vi "SwissSPAD Live_Image Histogram.vi"() -> ()   [LabVIEW 2021]
uses:
  Histograms/Histogram Bin Position.ctl
  SwissSPAD Live_Internal Data List.ctl
  SwissSPAD Live_Settings List.ctl
  SwissSPAD Live_Image Display Options.ctl
  Calc/Conditional Add 1.llb/Conditional Add 1 [I32].vi
  3eb8dcdc-dfa2-4210-84d8-37bed86b0045.vi/929807a6-00f9-4258-af09-20dfd637e3ca.vi
  3eb8dcdc-dfa2-4210-84d8-37bed86b0045.vi/52c6b4fa-501b-4af0-803b-8bab516ca5d3.vi
  3eb8dcdc-dfa2-4210-84d8-37bed86b0045.vi/d7237e10-35ab-4bcb-a0c6-4883c3f4c990.vi
  3eb8dcdc-dfa2-4210-84d8-37bed86b0045.vi/5fb5dd96-3b97-4592-ba56-58181c8e7105.vi
  3eb8dcdc-dfa2-4210-84d8-37bed86b0045.vi/8e13a849-a393-4484-9968-4af7b25c38d7.vi
  GUI/Dialog Window with Option.vi
  <vilib>/Analysis/baseanly.llb/Std Deviation and Variance.vi
  <vilib>/Utility/error.llb/Error Cluster From Error Code.vi
  Variant/Variant to Data/Variant to Data.lvlib
panel:
  in  "Cursor Update (Hidden)":bool
  in  "Stop (Hidden)":bool
  out "Image Histogram":cluster{"Axis":dbl[], "Histogram":dbl[]}(graph)
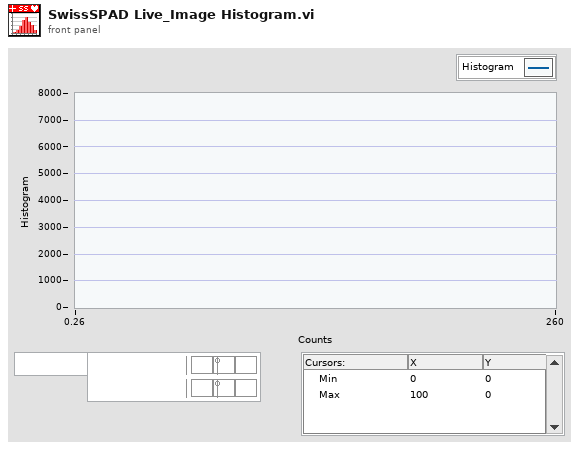
[diagram p1: front panel]
types:
  T1 = typedef "Histogram Bin Position.ctl" = enum16{"Left", "Center", "Right"}
  T2 = cluster{"Bin Size":dbl, "Min Value":dbl, "Max Value":dbl, "Filter NaN & Infinite Values":bool, "Frequency Plot":bool, "Align Bins":bool, "Bin Location":T1, "Project Outside Values":bool, "Max Histogram Size":i32}
  T3 = typedef "SwissSPAD Live_Internal Data List.ctl" = enum16{"Number of pending file saving tasks", "File Saving Tasks Information", "Current Image ROI Information", "# FPGA Reset Attempts", "Histogram Cursor Locations", "Histogram Window is Open"}
  T4 = typedef "SwissSPAD Live_Settings List.ctl" = enum16{"FPGA:Bottom Half", "FPGA:Top Half", "FPGA:Bottom Bitfile Path", "FPGA:Top Bitfile Path", "FPGA:Bottom Bitstream Version", "FPGA:Top Bitstream Version", "FPGA:Auto Reset FPGA", "FPGA:Bottom FPGA Serial Number", "FPGA:Top FPGA Serial Number", "FPGA:Detector PCB Version", "Acquisition Parameters:Microlens", "Acquisition Parameters:SS2 DAQ Parameters", "Acquisition Parameters:Gate Configuration Array", "Acquisition Parameters:SS3 DAQ Parameters", "Acquisition Parameters:Buffer Size (# 8-bit Gates)", "File Information:File Information", "File Information:# Datasets in Series", "File Information:Scrambled File Flag", "File Information:SS3 Gate Slip Correction", "File Information:SS3 Hot Pixel Mismatch Detection", "File Information:Delay between Datasets", "File Information:Save Sum of All Gates Preview", "Image Parameters:Image ROI Information", "Image Parameters:Image Binning Options", "Image Parameters:SS3 Displayed Image", "Image Parameters:Image Display Options", "Image Parameters:Use Histogram Cursors", "Image Parameter:FPGA Data to Display", "UI Settings:Histogram Bins Number", "UI Settings:Histogram Bin Size", "UI Settings:Use Image Display Options", "UI Settings:Verbose Settings", "UI Settings:Verbose Saving"}
  T5 = typedef "SwissSPAD Live_Image Display Options.ctl" = cluster{"Remove Screamers":bool, "Delta":sgl, "Equalize Histogram":bool, "Percentile":sgl, "Hot Pixel Mask Image":path, "Use Hot Pixel Mask":bool}
  T6 = typedef "Array Statistics.ctl" = cluster{"Mean":dbl, "Standard Deviation":dbl, "Max":dbl, "Min":dbl}
  T7 = typedef "LVCursorListTypeDef.ctl" = cluster{"Name":string, "Color":u32, "Style":u8, "Point Style":u8, "Name Visible":bool, "Allow Drag":bool, "Cursor Mode":u32, "Plot":i32, "Index":i32, "Position":cluster{"X":dbl, "Y":dbl}, "X Scale":u32, "Y Scale":u32, "Watch Plots":i32[], "Watch All Plots":bool, "Plot Area":i32, "Label Offset":cluster{"X":dbl, "Y":dbl}}[]
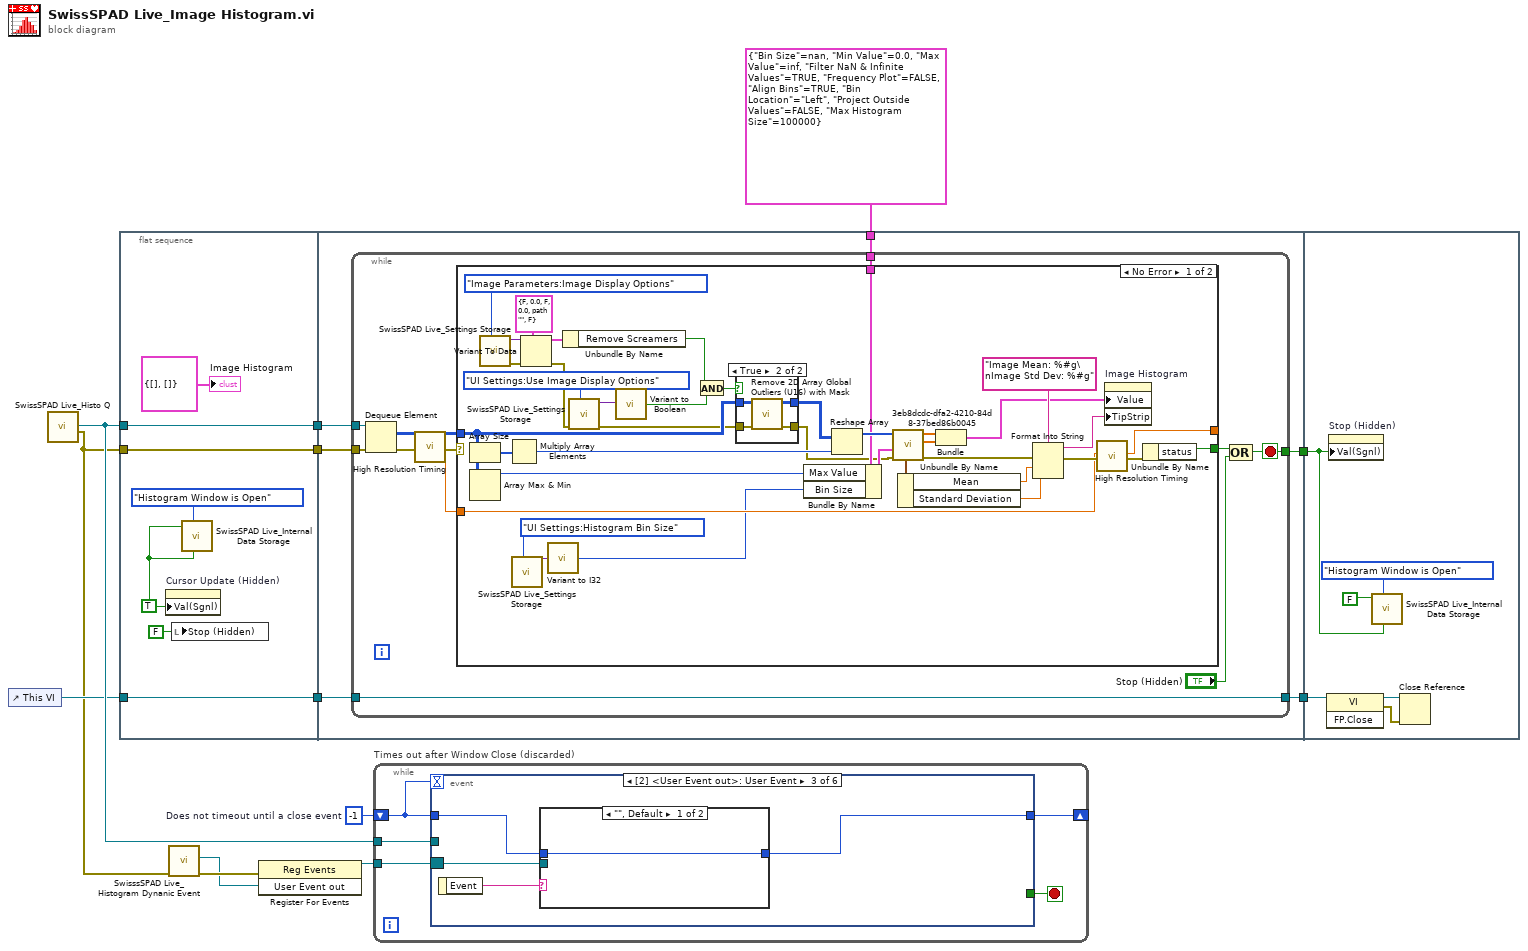
[diagram p0: block diagram]
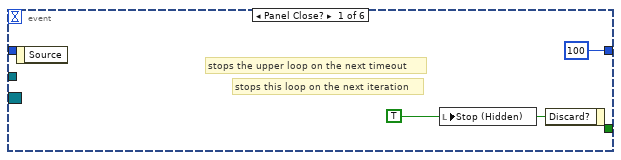
[diagram p2: hidden frame]
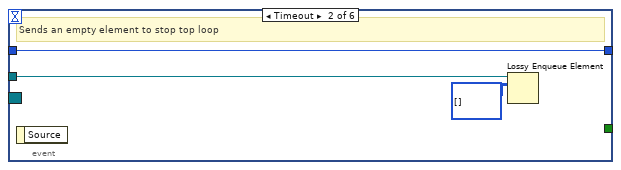
[diagram p3: hidden frame]
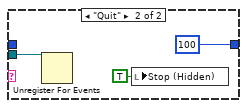
[diagram p4: hidden frame]
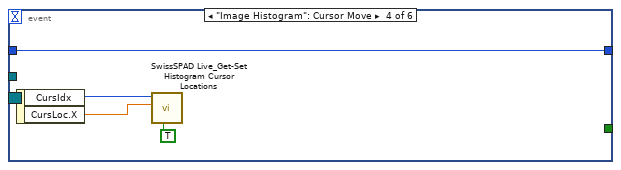
[diagram p5: hidden frame]
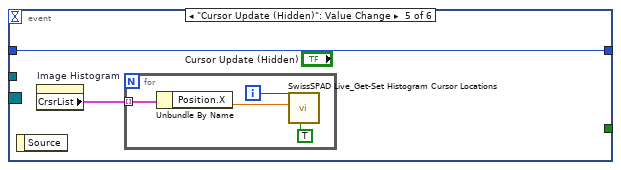
[diagram p6: hidden frame]
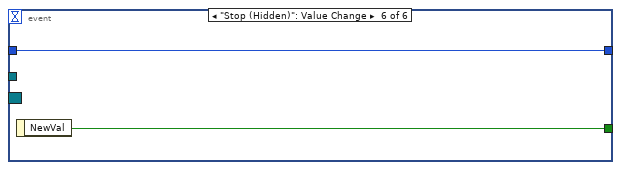
[diagram p7: hidden frame]
diagram:
  w11 = -1  # Does not timeout until a close event
  n1 = control-ref of="This VI"() -> (w6:refnum<vi>)
  n2 = call "SwissSPAD Live_Histo Q.vi"() -> ("error out"=w1:errorcluster, "SS2 Live Histo Q"=w8:refnum<queue>)  [unwired: 6 in]
  n3 = flat-sequence {
    tunnel: [w19] -> w10
    tunnel: w8 -> [w19]
    tunnel: [w18] -> w9
    tunnel: w1 -> [w18]
    tunnel: [w17] -> w7
    tunnel: w6 -> [w17]
    tunnel: [w26] -> w13
    tunnel: [w22] -> w12
    tunnel: w10 -> [w25]
    tunnel: w9 -> [w24]
    tunnel: w7 -> [w23]
    tunnel: T2 {"Bin Size"=nan, "Min Value"=0.0, "Max Value"=inf, "Filter NaN & Infinite Values"=TRUE, "Frequency Plot"=FALSE, "Align Bins"=TRUE, "Bin Location"=enum."Left", "Project Outside Values"=FALSE, "Max Histogram Size"=100000} ("Histogram Options") -> [w21]
    tunnel: w13 -> [w83]
    tunnel: w12 -> [w87]
    frame #0 {
      w16 = TRUE ("Value (Signaling)")
      n4 = property on="Cursor Update (Hidden)" class="Bool (strict)"("Val(Sgnl)"=w16) -> ()  [unwired: 2 in, 2 out]
      n5 = local write "Stop (Hidden)"(FALSE ("Stop")) -> ()
      n6 = call "SwissSPAD Live_Internal Data Storage.vi"("Get(F)/Set"=w16, "SS2 Live Data"=SwissSPAD_Live_Internal_Data_List."Histogram Window is Open", "Variant"=w16) -> ()  [unwired: 6 in, 3 out]
      "Image Histogram" <- cluster{"Axis":dbl[], "Histogram":dbl[]} {"Axis"=[], "Histogram"=[]} ("Image Histogram")
    }
    frame #1 {
      n7 = while {
        tunnel: [w33] -> w26
        tunnel: w25 -> [w32]
        tunnel: w24 -> [w31]
        tunnel: w23 -> [w30]
        tunnel: [w30] -> w22
        tunnel: w21 -> [w27]
        stop <- w33 stop-if-true
        n8 = Dequeue Element(queue=w32, error in (no error)=w31) -> (element=w36:u16[][], error out=w37:errorcluster)  [unwired: 1 in, 2 out]
        n9 = call "High Resolution Timing.vi"("Error In"=w37) -> ("elapsed (relative) seconds"=w28:dbl, "Error Out"=w29:errorcluster)  [unwired: 16 in, 1 out]
        n10 = case shown="No Error" w29 {
          tunnel: w36 -> [w45 _]
          tunnel: [w74 _] -> w35
          tunnel: w28 -> [w58 _]
          tunnel: [w57 _] -> _
          tunnel: w27 -> [w56 _]
          frame No Error {
            n11 = Array Size(array=w45) -> (size(s)=w73:i32[])
            n12 = Array Max & Min(array=w45) -> (max value=w61:u16)  [unwired: 3 out]
            n13 = call "SwissSPAD Live_Settings Storage.vi"("Settings List"=SwissSPAD_Live_Settings_List."Image Parameters:Image Display Options") -> ("Error Out"=w50:errorcluster, "Variant Data out"=w51:variant)  [unwired: 9 in]
            n14 = Multiply Array Elements(1:w73) -> (0:w72:i32)
            n15 = call "SwissSPAD Live_Settings Storage.vi"("Settings List"=SwissSPAD_Live_Settings_List."UI Settings:Histogram Bin Size") -> ("Variant Data out"=w54:variant)  [unwired: 9 in, 1 out]
            n16 = Variant To Data(error in=w50, type=T5 {"Remove Screamers"=FALSE, "Delta"=0.0, "Equalize Histogram"=FALSE, "Percentile"=0.0, "Hot Pixel Mask Image"=path "", "Use Hot Pixel Mask"=FALSE} ("Image Display Options"), Variant=w51) -> (data=w48:T5, error out=w43:errorcluster)
            n17 = call "Variant to I32.vi"("Variant"=w54) -> ("Value"=w38:i32)  [unwired: 8 in]
            n18 = Unbundle By Name(w48) -> ("Remove Screamers"=w47:bool)
            n19 = call "SwissSPAD Live_Settings Storage.vi"("Settings List"=SwissSPAD_Live_Settings_List."UI Settings:Use Image Display Options", "Error In"=w43) -> ("Error Out"=w40:errorcluster, "Variant Data out"=w42:variant)  [unwired: 8 in]
            n20 = call "Variant to Boolean.vi"("Variant"=w42) -> ("Value"=w41:bool)  [unwired: 8 in]
            n21 = And(x=w47, y=w41) -> (x .and. y?=w46:bool)
            n22 = case shown="True" w46 {
              tunnel: [w77 w81] -> w53
              tunnel: w40 -> [w76 w80]
              tunnel: w45 -> [w77 w79]
              tunnel: [w76 w78] -> w39
              frame False {
              }
              frame True {
                n23 = call "Remove 2D Array Global Outliers (U16) with Mask.vi"("Error In"=w80, "2D Array in"=w79) -> ("Error Out"=w78:errorcluster, "2D Array out"=w81:u16[][])  [unwired: 6 in, 2 out]
              }
            }
            n24 = Bundle By Name(cluster=w56, "Max Value"=w61, "Bin Size"=w38) -> (w60:T2)
            n25 = Reshape Array(w53, w72) -> (w71:u16[])
            n26 = call "3eb8dcdc-dfa2-4210-84d8-37bed86b0045.vi"("Error In"=w39, "Histogram Options"=w60, "Array"=w71) -> ("Error Out"=w70:errorcluster, "Array Statistics"=w69:T6, "Histogram"=w65:dbl[], "Axis"=w66:dbl[])  [unwired: 4 in, 1 out]
            n27 = Unbundle By Name(w69) -> ("Mean"=w68:dbl, "Standard Deviation"=w67:dbl)
            n28 = Bundle("Axis"=w66, "Histogram"=w65) -> (w63:cluster{"Axis":dbl[], "Histogram":dbl[]})  [unwired: 1 in]
            n29 = Format Into String(format string="Image Mean: %#g\nImage Std Dev: %#g", error in=w70, w68, w67) -> (resulting string=w62:string, error out=w64:errorcluster)  [unwired: 1 in]
            n30 = call "High Resolution Timing.vi"("relative seconds (NaN)"=w58, "Error In"=w64) -> ("elapsed (relative) seconds"=w57:dbl, "Error Out"=w59:errorcluster)  [unwired: 15 in, 1 out]
            n31 = property on="Image Histogram" class="XYGraph (strict)"("Value"=w63, "TipStrip"=w62) -> ()  [unwired: 2 in, 2 out]
            n32 = Unbundle By Name(w59) -> ("status"=w74:bool)
          }
          frame Error {
          }
        }
        n33 = Compound Arithmetic op=OR(w35, "Stop (Hidden)") -> (w33:bool)
      }
    }
    frame #2 {
      n34 = invoke class="VI" method="FP.Close"(reference=w87) -> (reference out=w86:refnum<vi>, error out=w85:errorcluster)  [unwired: 2 in, 1 out]
      n35 = property on="Stop (Hidden)" class="Bool (strict)"("Val(Sgnl)"=w83) -> ()  [unwired: 2 in, 2 out]
      n36 = call "SwissSPAD Live_Internal Data Storage.vi"("Get(F)/Set"=w83, "SS2 Live Data"=SwissSPAD_Live_Internal_Data_List."Histogram Window is Open", "Variant"=FALSE) -> ()  [unwired: 6 in, 3 out]
      n37 = Close Reference(reference=w86, error in (no error)=w85) -> ()  [unwired: 1 out]
    }
  }
  n38 = call "SwisssSPAD Live_Histogram Dynanic Event.vi"("error in"=w1) -> ("error out"=w3:errorcluster, "User Event out"=w2:refnum<user-event>)  [unwired: 9 in]
  n39 = register-events(error in=w3, w2) -> (reference out=w4:refnum<event-registration>)  [unwired: 1 in, 1 out]
  n40 = while "Times out after Window Close (discarded)" {
    tunnel: w8 -> [w91]
    shift-right: [w90] -> _
    shift-left: w11 -> [w89]
    tunnel: w4 -> [w88]
    stop <- w92 stop-if-true
    n41 = event shown="[2] <User Event out>: User Event" {
      selector: w88 -> [_ _ w99 _ _ _]
      dyn-events: _ -> [_ _ _ _ _ _]
      timeout: w89 -> [_ _ _ _ _ _]
      tunnel: [_ _ _ _ _ w117] -> w92
      tunnel: w91 -> [_ w97 _ _ _ _]
      tunnel: [100 w96 w100 w106 w110 w116] -> w90
      tunnel: w89 -> [_ w96 w98 w106 w110 w116]
      event Panel Close? {
        w93 = TRUE ("Discard?")
        # "stops the upper loop on the next timeout"
        # "stops this loop on the next iteration"
        n42 = event-data() -> ()  [unwired: 1 in, 1 out]
        n43 = local write "Stop (Hidden)"(w93) -> ()
        n44 = event-data("Discard?"=w93) -> ()  [unwired: 1 in, 1 out]
      }
      event Timeout {
        # "Sends an empty element to stop top loop"
        n45 = event-data() -> ()  [unwired: 1 in, 1 out]
        n46 = Lossy Enqueue Element(queue=w97, element=u16[][] []) -> ()  [unwired: 1 in, 4 out]
      }
      event User Event {
        n47 = event-data() -> ("Event"=w101:string)  [unwired: 1 in]
        n48 = case shown="\"\", Default" w101 {
          tunnel: [w102 100] -> w100
          tunnel: w99 -> [_ w103]
          tunnel: w98 -> [w102 _]
          frame "", Default {
          }
          frame "Quit" {
            n49 = Unregister For Events(event registration refnum=w103) -> ()  [unwired: 1 in, 1 out]
            n50 = local write "Stop (Hidden)"(TRUE ("Discard?")) -> ()
          }
        }
      }
      event "Image Histogram": Cursor Move {
        n51 = event-data() -> ("CursIdx"=w109:i32, "CursLoc.X"=w108:dbl)  [unwired: 1 in]
        n52 = call "SwissSPAD Live_Get-Set Histogram Cursor Locations.vi"("Get (F)/Set"=TRUE ("Get/Set"), "X"=w108, "CursIdx"=w109) -> ()  [unwired: 6 in, 3 out]
      }
      event "Cursor Update (Hidden)": Value Change {
        n53 = event-data() -> ()  [unwired: 1 in, 1 out]
        n54 = property on="Image Histogram" class="XYGraph (strict)"() -> ("CrsrList"=w111:T7)  [unwired: 2 in, 2 out]
        n55 = for {
          tunnel: w111 -> [w114] mode=indexing
          i -> [w112]
          n56 = Unbundle By Name(w114) -> ("Position.X"=w113:dbl)
          n57 = call "SwissSPAD Live_Get-Set Histogram Cursor Locations.vi"("Get (F)/Set"=TRUE ("Get/Set"), "X"=w113, "CursIdx"=w112) -> ()  [unwired: 6 in, 3 out]
        }
      }
      event "Stop (Hidden)": Value Change {
        n58 = event-data() -> ("NewVal"=w117:bool)  [unwired: 1 in]
      }
    }
  }
